vi "Parse Message Payload.vi"(8 "error in":errorcluster, 11 "TCP Message In":string) -> (0 "error out":errorcluster, 3 "Parsed Message":T1)   [LabVIEW 2018]
uses:
  Button Class/TCP Message Payload.ctl
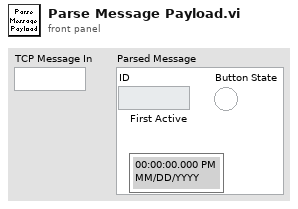
[diagram p1: front panel]
types:
  T1 = typedef "TCP Message Payload.ctl" = cluster{"ID":string, "First Active":timestamp, "Button State":bool}
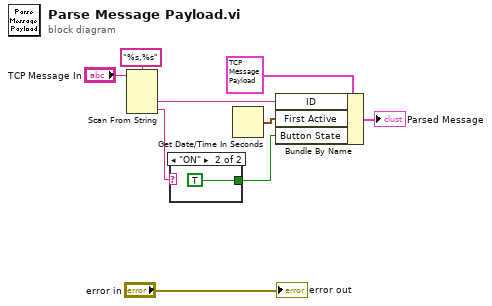
[diagram p0: block diagram]
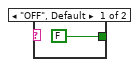
[diagram p2: hidden frame]
diagram:
  n1 = Scan From String(format string="%s,%s", input string="TCP Message In") -> (output 1=w9:string, output 2=w4:string)  [unwired: 4 in, 3 out]
  n2 = case shown="\"ON\"" w4 {
    tunnel: [FALSE TRUE] -> w2
    frame "OFF", Default {
    }
    frame "ON" {
    }
  }
  n3 = Get Date/Time In Seconds() -> (seconds since 1Jan1904=w3:timestamp)
  n4 = Bundle By Name(cluster=T1 {"ID"="", "First Active"=timestamp(0 s since 1904-01-01), "Button State"=FALSE} ("Message Payload"), "ID"=w9, "First Active"=w3, "Button State"=w2) -> (→"Parsed Message":T1)
  "error out" <- "error in"
